vi "UEvent_SET_INTERNAL_EXTERNAL_POWER_SOURCE.vi"(6 "Ex/Int PW":T1(ring), 8 "Ext PW Vol Monitor":bool, 9 "USB":tag, 10 "Value":T2, 11 "Refnum in":refnum<k21>) -> (0 "External Voltage HIGH":bool, 1 "Battery_Voltage":dbl, 2 "DUT_Voltage":dbl, 3 "Refnum out":refnum<k21>)   [LabVIEW 2015]
uses:
  Range_Shunt_selector.ctl
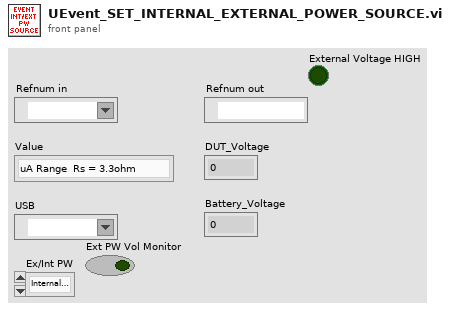
[diagram p1: front panel]
types:
  T1 = enum16{"Internal PW Source", "External PW Source"}
  T2 = typedef "Range_Shunt_selector.ctl" = enum16{"uA Range  Rs = 3.3ohm", "mA Range Rs = 3.3Ohm", "mA Range Rs = 1Ohm", "mA Range Rs = 1Ohm - X2"}
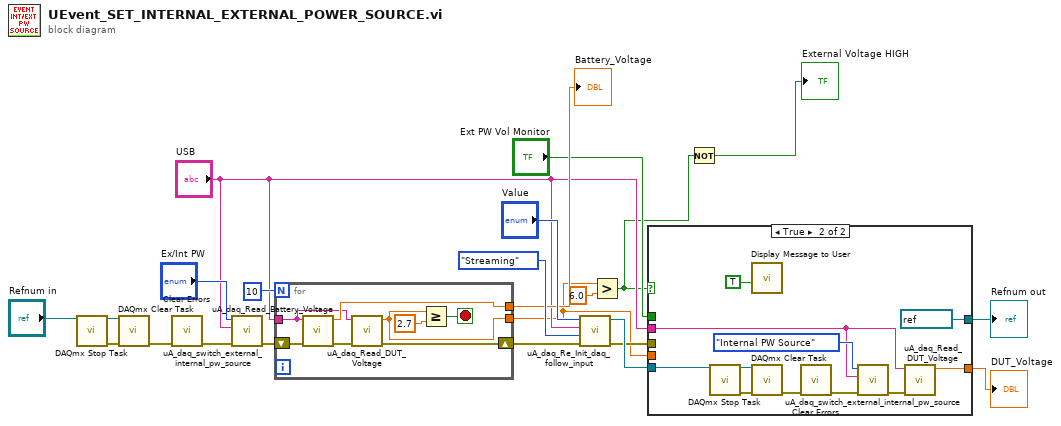
[diagram p0: block diagram]
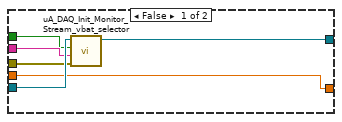
[diagram p2: hidden frame]
diagram:
  n1 = call <vilib>:"DAQmx Stop Task.vi"("task/channels in"="Refnum in") -> ("task out"=w16:refnum<k21>, "error out"=w13:errorcluster)  [unwired: 13 in]
  n2 = call <vilib>:"DAQmx Clear Task.vi"("task in"=w16, "error in"=w13) -> ("error out"=w14:errorcluster)  [unwired: 13 in]
  n3 = call <vilib>:"Clear Errors.vi"("error in (no error)"=w14) -> ("error out"=w19:errorcluster)  [unwired: 5 in, 1 out]
  n4 = call "uA_daq_switch_external_internal_pw_source.vi"("error in"=w19, "USB DAQ"="USB", "Ex/Int PW"="Ex/Int PW") -> ("error out"=w12:errorcluster)  [unwired: 8 in]
  n5 = for {
    N: 10 -> [_]
    tunnel: [w23] -> w3
    tunnel: [w28] -> w17
    tunnel: "USB" -> [w27]
    shift-right: [w30] -> w22
    shift-left: w12 -> [w26]
    stop <- w24 stop-if-true
    n6 = call "uA_daq_Read_Battery_Voltage.vi"("error in"=w26, "USB DAQ"=w27) -> ("error out"=w29:errorcluster, "Battery_Voltage"=w28:dbl)  [unwired: 8 in]
    n7 = call "uA_daq_Read_DUT_Voltage.vi"("error in"=w29, "USB DAQ"=w27) -> ("error out"=w30:errorcluster, "DUT_Voltage"=w23:dbl)  [unwired: 8 in]
    n8 = Greater Or Equal?(x=w23, y=2.7) -> (x >= y?=w24:bool)
  }
  "Battery_Voltage" <- w17
  n9 = call "uA_daq_Re_Init_daq_follow_input.vi"("error in (no error)"=w22, "Acquire Mode"=enum16{"Streaming", "Read All", "Stop"}."Streaming", "USB"="USB", "Range_shunt"="Value") -> ("error out"=w6:errorcluster, "Refnum out"=w8:refnum<k21>)  [unwired: 6 in]
  n10 = Greater?(x=w3, y=6.0) -> (0:w2:bool)
  n11 = case shown="True" w2 {
    tunnel: "USB" -> [w33 w39]
    tunnel: w8 -> [w36 w42]
    tunnel: [w35 refnum<k21> "Stop" ("Refnum out")] -> w7
    tunnel: w6 -> [w34 _]
    tunnel: "Ext PW Vol Monitor" -> [w32 _]
    tunnel: [w31 w37] -> w4
    tunnel: w3 -> [w31 _]
    frame False {
      n12 = call "uA_DAQ_Init_Monitor_Stream_vbat_selector.vi"("error in (no error)"=w34, "USB"=w33, "Ext PW Vol Monitor"=w32, "Refnum in"=w36) -> ("Refnum out"=w35:refnum<k21>)  [unwired: 6 in, 1 out]
    }
    frame True {
      n13 = call <vilib>:"DAQmx Stop Task.vi"("task/channels in"=w42) -> ("task out"=w45:refnum<k21>, "error out"=w47:errorcluster)  [unwired: 13 in]
      n14 = call "Display Message to User"("Enable"=TRUE) -> ()  [unwired: 9 in, 2 out]
      n15 = call <vilib>:"DAQmx Clear Task.vi"("task in"=w45, "error in"=w47) -> ("error out"=w46:errorcluster)  [unwired: 13 in]
      n16 = call <vilib>:"Clear Errors.vi"("error in (no error)"=w46) -> ("error out"=w44:errorcluster)  [unwired: 5 in, 1 out]
      n17 = call "uA_daq_switch_external_internal_pw_source.vi"("error in"=w44, "USB DAQ"=w39, "Ex/Int PW"=T1."Internal PW Source") -> ("error out"=w38:errorcluster)  [unwired: 8 in]
      n18 = call "uA_daq_Read_DUT_Voltage.vi"("error in"=w38, "USB DAQ"=w39) -> ("DUT_Voltage"=w37:dbl)  [unwired: 8 in, 1 out]
    }
  }
  "Refnum out" <- w7
  "DUT_Voltage" <- w4
  n19 = Not(x=w2) -> (.not. x?=→"External Voltage HIGH":bool)
